vi "Get Grayscale Value.vi"(2 "input color":u32(colorbox)) -> (5 "grayscale value":u8)   [LabVIEW 2021, in "lv_icon.lvlib"]
doc: "Determine the gray scale value of a color."
uses:
  <vilib>/LabVIEW Icon API/lv_icon/lv_icon.lvlib
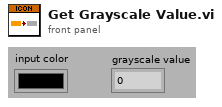
[diagram p1: front panel]
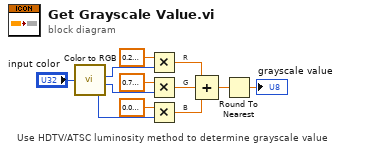
[diagram p0: block diagram]
diagram:
  # "B"
  # "G"
  # "R"
  # "Use HDTV/ATSC luminosity method to determine grayscale value"
  n1 = call <vilib>:"Color to RGB.vi"("Color"="input color") -> ("R"=w1:u8, "G"=w2:u8, "B"=w3:u8)  [unwired: 1 out]
  n2 = Multiply(x=sgl 0.2126, y=w1) -> (x*y=w9:sgl)
  n3 = Multiply(x=sgl 0.7152, y=w2) -> (x*y=w7:sgl)
  n4 = Multiply(x=sgl 0.0722, y=w3) -> (x*y=w8:sgl)
  n5 = Compound Arithmetic op=ADD(w9, w7, w8) -> (w6:sgl)
  n6 = Round To Nearest(number=w6) -> (nearest integer value=→"grayscale value":sgl)
